vi "Read_FV_Data.vi"(8 "error in (no error)":errorcluster, 9 "RFID":string, 10 "View":bool, 11 "MS SQL Connection":T1) -> (0 "error out":errorcluster, 1 "Enable?":bool, 2 "spreadsheet string":string, 3 "Report":string[][](array[string]), 4 "REsult":T2, 5 "Final View Barcode":string, 6 "All Status":string[](array[string]), 7 "ASR Barcode":string)   [LabVIEW 2020]
uses:
  Controls/FV_Status.ctl
  <vilib>/addons/database/Connection.llb/Conn ObjectReference.ctl
  MS SQL/MS_Global.vi
  <vilib>/ethernetip/ethernetip.llb/EthernetIP Tag Write DINT.vi
  <userlib>/_OpenG.lib/string/string.llb/To Proper Case (String)__ogtk.vi
  <vilib>/addons/database/Connection.llb/Conn Execute.vi
  <vilib>/addons/database/Recordset.llb/Rec Fetch Recordset Data (R).vi
  <vilib>/addons/database/Recordset.llb/Rec Destroy - Connection.vi
  <vilib>/addons/database/_DB Variant To Data/Database Variant To Data.xnode
  <vilib>/addons/database/NI_Database_API.lvlib
  <vilib>/ethernetip/ethernetip.lvlib
panel:
  out "All Result":bool[](array[boolean])
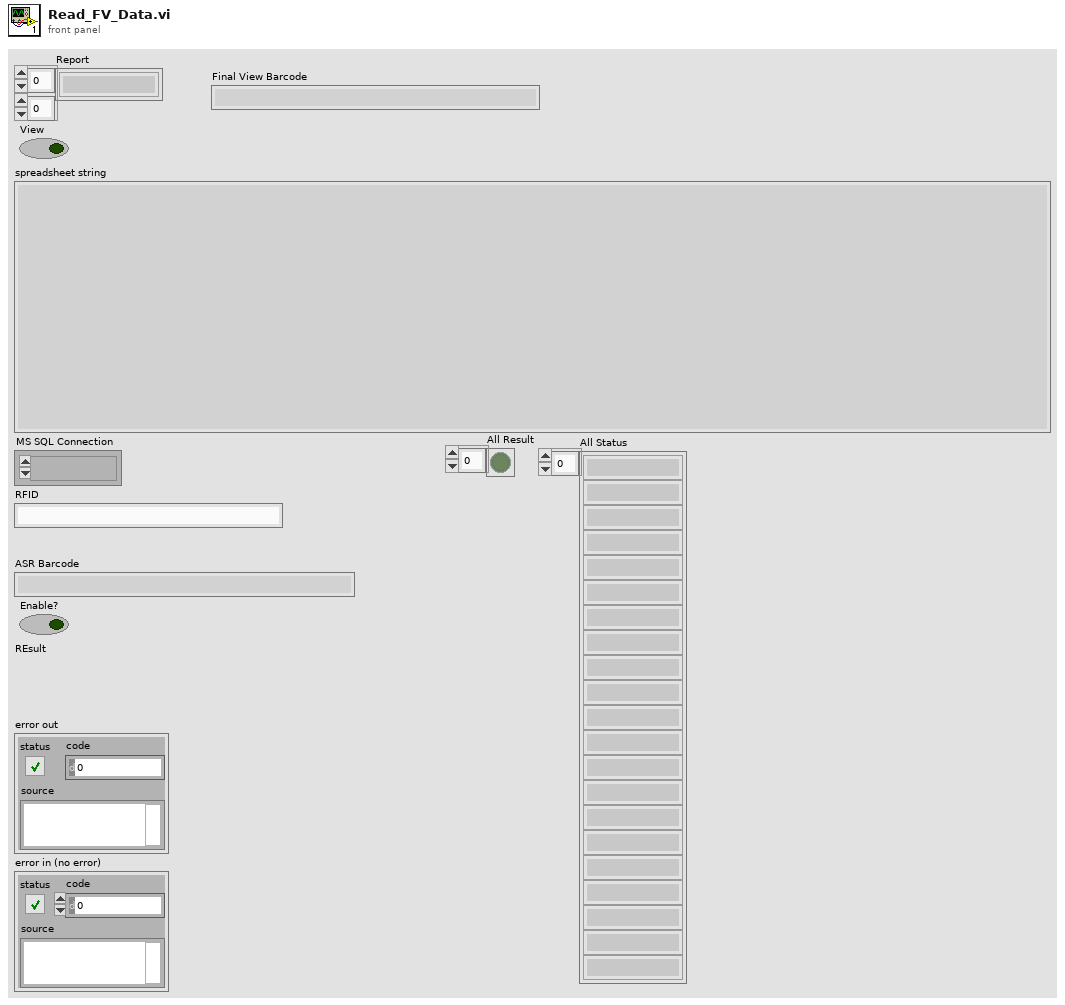
[diagram p1: front panel]
types:
  T1 = typedef "NI_Database_API.lvlib/Conn ObjectReference.ctl" = refnum<k1>
  T2 = typedef "FV_Status.ctl" = u16
  T3 = typedef "TD SQL.ctl" = cluster{"MS SQL Connection":T1, "UDL File":path, "Time":string, "DCODE":string, "WIP+1":i64, "MC No?":i32, "POKAYOKE?":bool, "Expected Result":string, "Result [Status]":string, "Clock":dbl, "RFID":string, "WIP Queue":refnum<queue>, "TS Parameter":T4, "Data_Queue":refnum<queue>[], "RFID Serial No.":string}
  T4 = typedef "TS_Parameter.ctl" = cluster{"ProfitCenterCode":string, "LineCode":string, "WorkOrderNumber":string, "Model":string, "Model_with_Prefix":string, "VendorCode":string, "SetParameterDateCode":string, "PokaYoke":i32, "Target":i32, "Live_DateCode":string, "CustomerPartNumber":string, "Hand":string, "sBarcode":bool, "FCA":i32, "Ent_Stamp":timestamp, "STS_CD":dbl}
  T5 = typedef "NI_Database_API.lvlib/Rec ObjectReference.ctl" = refnum<k1>
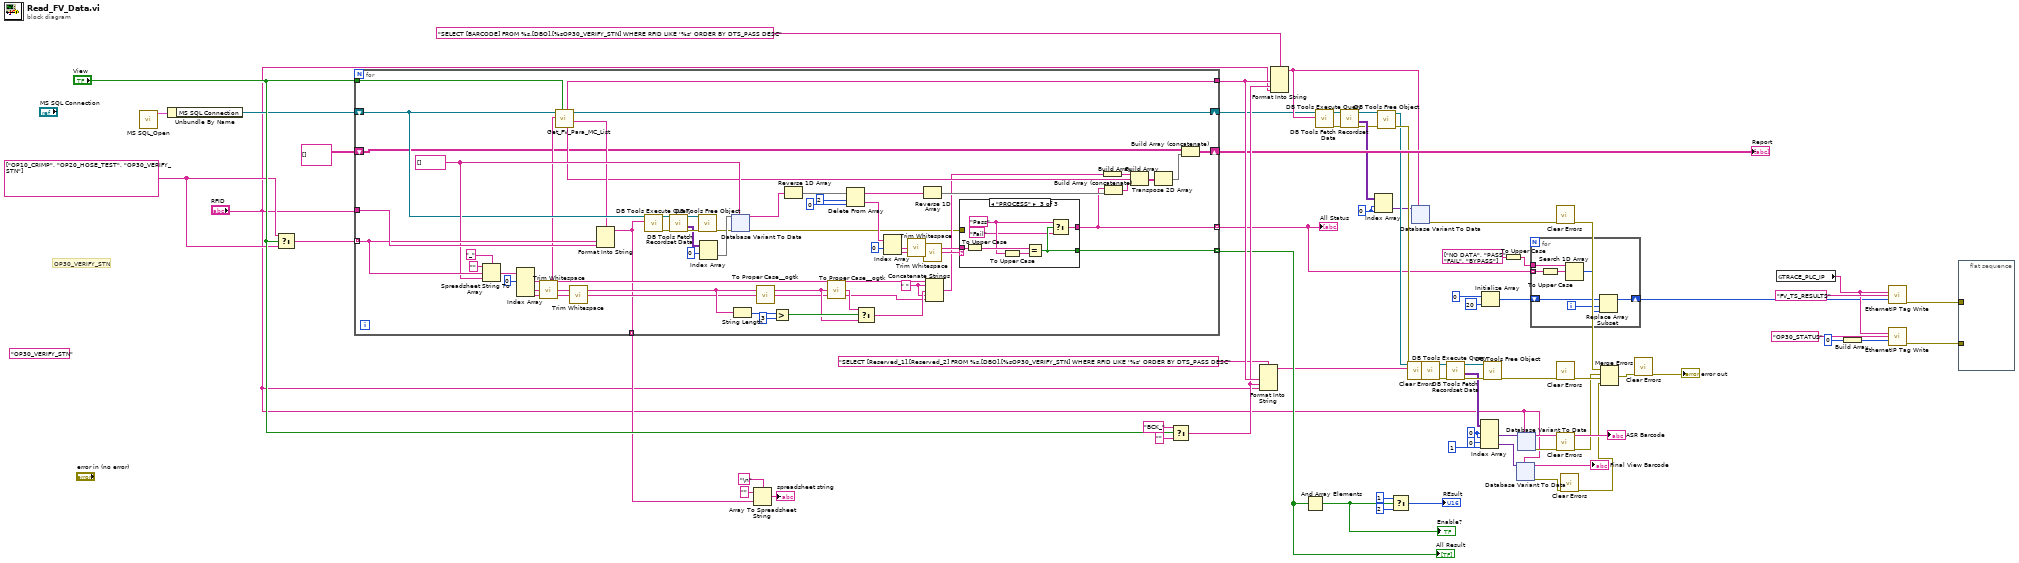
[diagram p0: block diagram]
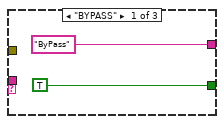
[diagram p2: hidden frame]
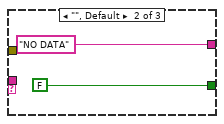
[diagram p3: hidden frame]
diagram:
  w46 = 0 ("index (row)")
  w41 = 0 ("index (row)")
  (unwired) "OP30_VERIFY_STN" ("String")
  w9 = string[] ["OP10_CRIMP", "OP20_HOSE_TEST", "OP30_VERIFY_STN"] ("tables 2")
  # "OP30_VERIFY_STN"
  n1 = call "MS SQL_Open.vi"() -> ("Ref Out"=w10:T3)  [unwired: 9 in, 2 out]
  n2 = Unbundle By Name(w10) -> ("MS SQL Connection"=w28:T1)
  n3 = Select(t=w9, s="View", f=w9) -> (s? t:f=w66:string[])
  n4 = for {
    tunnel: w66 -> [w120] mode=indexing
    tunnel: "RFID" -> [w128]
    tunnel: [w121] -> w57 mode=indexing
    tunnel: [w86] -> w25 mode=indexing
    shift-right: [w102] -> w37
    shift-left: w28 -> [w103]
    tunnel: [w75] -> w60 mode=indexing
    shift-right: [w95] -> w65
    shift-left: string[][] [] ("appended array") -> [w97]
    tunnel: "View" -> [w85]
    tunnel: [w84] -> w72
    w81 = " " ("string")
    w119 = string[] [] ("tables 2")
    n5 = Spreadsheet String To Array(delimiter (Tab)="_", format string="", spreadsheet string=w120, array type (2D Dbl)=w119) -> (array=w112:string[])
    n6 = Index Array(array=w112, index #1=0 ("index")) -> (element #1=w101:string, element #3=w113:string, element #4=w80:string)  [unwired: 3 in, 1 out]
    n7 = call <vilib>:"Trim Whitespace.vi"("string"=w113) -> ("trimmed string"=w107:string)  [unwired: 1 in]
    n8 = call "Get_FV_Para_MC_List.vi"("View"=w85, "Machine No."=w101, "Refnum in"=w103) -> ("Search Queary"=w100:string, "Refnum out"=w102:T1, "Column Display"=w99:string[], "Table"=w84:string)  [unwired: 3 in, 2 out]
    n9 = call <vilib>:"Trim Whitespace.vi"("string"=w80) -> ("trimmed string"=w83:string)  [unwired: 1 in]
    n10 = Format Into String(format string=w100, w120, w128) -> (resulting string=w75:string)  [unwired: 2 in, 1 out]
    n11 = call-poly <vilib>:"DB Tools Execute Query.vi"("SQL query"=w75, "connection reference"=w103) -> ("error out"=w126:errorcluster, "recordset reference"=w127:T5)  [unwired: 6 in]
    n12 = call-poly <vilib>:"DB Tools Fetch Recordset Data.vi"("error in (no error)"=w126, "recordset reference"=w127) -> ("error out"=w78:errorcluster, "recordset data"=w76:variant[][], "recordset reference out"=w79:T5)  [unwired: 3 in]
    n13 = call-poly <vilib>:"DB Tools Free Object.vi"("error in (no error)"=w78, "recordset reference"=w79) -> ("error out"=w73:errorcluster)  [unwired: 8 in, 1 out]
    n14 = Index Array(array=w76, index (row)=0) -> (element=w124:variant[])  [unwired: 1 in]
    n15 = xnode "Database Variant To Data"("database variant"=w124, "error in (no error)"=w73, "type"=w119) -> ("data"=w123:string[], "error out"=w74:errorcluster)
    n16 = String Length(string=w107) -> (length=w111:i32)
    n17 = call-poly <userlib>:"To Proper Case__ogtk.vi"("string"=w83) -> ("proper case string"=w82:string)  [unwired: 4 in]
    n18 = Greater?(x=w111, y=3) -> (0:w109:bool)
    n19 = Reverse 1D Array(array=w123) -> (reversed array=w93:string[])
    n20 = call-poly <userlib>:"To Proper Case__ogtk.vi"("string"=w107) -> ("proper case string"=w108:string)  [unwired: 4 in]
    n21 = Delete From Array(array=w93, length=2, index=0) -> (deleted portion=w91:string[], array with subset deleted=w89:string[])
    n22 = Select(t=w108, s=w109, f=w107) -> (s? t:f=w106:string)
    n23 = Index Array(array=w91, index #1=0 ("index (row)")) -> (element #1=w115:string, element #2=w114:string)  [unwired: 1 in]
    n24 = call <vilib>:"Trim Whitespace.vi"("string"=w115) -> ("trimmed string"=w105:string)  [unwired: 1 in]
    n25 = call <vilib>:"Trim Whitespace.vi"("string"=w114) -> ("trimmed string"=w104:string)  [unwired: 1 in]
    n26 = Reverse 1D Array(array=w89) -> (reversed array=w87:string[])
    n27 = Concatenate Strings(w101, w81, w106, w81, w82) -> (w77:string)
    n28 = case shown="\"PROCESS\"" w104 {
      tunnel: w105 -> [_ _ w139]
      tunnel: [TRUE FALSE w137] -> w121
      tunnel: ["ByPass" ("String") "NO DATA" ("String") w136] -> w86
      tunnel: w74 -> [_ _ _]
      frame "BYPASS" {
      }
      frame "", Default {
      }
      frame "PROCESS" {
        w135 = "Pass" ("y")
        n29 = To Upper Case(1:w139) -> (0:w138:string)
        n30 = To Upper Case(1:w135) -> (0:w133:string)
        n31 = Equal?(x=w138, y=w133) -> (x = y?=w137:bool)
        n32 = Select(t=w135, s=w137, f="Fail" ("t")) -> (s? t:f=w136:string)
      }
    }
    n33 = Build Array(w77) -> (w98:string[])
    n34 = Build Array (concatenate)(w86, w87) -> (w88:string[])
    n35 = Build Array(w98, w99, w88) -> (w96:string[][])
    n36 = Transpose 2D Array(2D array=w96) -> (transposed array=w94:string[][])
    n37 = Build Array (concatenate)(w97, w94) -> (w95:string[][])
  }
  "Report" <- w65
  "All Result" <- w57
  "All Status" <- w25
  n38 = Array To Spreadsheet String(delimiter (Tab)="\n", array=w60, 3:"" ("format string")) -> (spreadsheet string=→"spreadsheet string":string)
  n39 = Select(t="BCK_", s="View", f="") -> (s? t:f=w71:string)
  n40 = Format Into String(format string="SELECT [Reserved_1],[Reserved_2] FROM %s.[DBO].[%sOP30_VERIFY_STN] WHERE RFID LIKE '%s' ORDER BY DTS_PASS DESC" ("String"), w72, w71, "RFID") -> (resulting string=w55:string)  [unwired: 2 in, 1 out]
  n41 = Format Into String(format string="SELECT [BARCODE] FROM %s.[DBO].[%sOP30_VERIFY_STN] WHERE RFID LIKE '%s' ORDER BY DTS_PASS DESC" ("String"), w72, w71, "RFID") -> (resulting string=w44:string)  [unwired: 2 in, 1 out]
  n42 = And Array Elements(Boolean array=w57) -> (logical AND=w18:bool)
  "Enable?" <- w18
  n43 = call-poly <vilib>:"DB Tools Execute Query.vi"("SQL query"=w44, "connection reference"=w37) -> ("error out"=w35:errorcluster, "recordset reference"=w36:T5)  [unwired: 6 in]
  n44 = call-poly <vilib>:"DB Tools Fetch Recordset Data.vi"("error in (no error)"=w35, "recordset reference"=w36) -> ("error out"=w38:errorcluster, "recordset data"=w40:variant[][], "recordset reference out"=w39:T5)  [unwired: 3 in]
  n45 = Index Array(array=w40, index (row)=w41, index (col)=w41) -> (element=w42:variant)
  n46 = call-poly <vilib>:"DB Tools Free Object.vi"("error in (no error)"=w38, "recordset reference"=w39) -> ("error out"=w53:errorcluster, "connection reference"=w52:T1)  [unwired: 8 in]
  n47 = Select(t=T2 1 ("Over all Status"), s=w18, f=T2 2) -> (s? t:f=→"REsult":T2)
  n48 = call <vilib>:"Clear Errors.vi"("error in (no error)"=w53) -> ("error out"=w8:errorcluster)  [unwired: 5 in, 1 out]
  n49 = xnode "Database Variant To Data"("database variant"=w42, "type"=w44) -> ("error out"=w32:errorcluster)  [unwired: 1 in, 1 out]
  n50 = call-poly <vilib>:"DB Tools Execute Query.vi"("error in (no error)"=w8, "SQL query"=w55, "connection reference"=w52) -> ("error out"=w51:errorcluster, "recordset reference"=w50:T5)  [unwired: 5 in]
  n51 = call-poly <vilib>:"DB Tools Fetch Recordset Data.vi"("error in (no error)"=w51, "recordset reference"=w50) -> ("error out"=w49:errorcluster, "recordset data"=w47:variant[][], "recordset reference out"=w48:T5)  [unwired: 3 in]
  n52 = Index Array(array=w47, index (row) #1=w46, index (col) #1=w46, index (row) #2=0 ("index (row)"), index (col) #2=1 ("disabled index (col)")) -> (element #1=w45:variant, element #2=w5:variant)
  n53 = Initialize Array(0 ("index of element"), 20 ("dimension size")) -> (w15:i32[])
  n54 = call-poly <vilib>:"DB Tools Free Object.vi"("error in (no error)"=w49, "recordset reference"=w48) -> ("error out"=w34:errorcluster)  [unwired: 8 in, 1 out]
  n55 = To Upper Case(1:string[] ["NO DATA", "PASS", "FAIL", "BYPASS"] ("Array")) -> (0:w11:string[])
  n56 = xnode "Database Variant To Data"("database variant"=w5, "type"="RFID") -> ("data"=→"Final View Barcode":string, "error out"=w2:errorcluster)  [unwired: 1 in]
  n57 = xnode "Database Variant To Data"("database variant"=w45, "type"="RFID") -> ("data"=→"ASR Barcode":string, "error out"=w33:errorcluster)  [unwired: 1 in]
  n58 = for {
    tunnel: w25 -> [w184] mode=indexing
    shift-right: [w179] -> w14
    shift-left: w15 -> [w182]
    tunnel: w11 -> [w178]
    i -> [w181]
    n59 = To Upper Case(1:w184) -> (0:w183:string)
    n60 = Search 1D Array(1D array=w178, element=w183) -> (index of element=w180:i32)  [unwired: 1 in]
    n61 = Replace Array Subset(array=w182, new element=w180, index=w181) -> (w179:i32[])
  }
  n62 = call <vilib>:"Clear Errors.vi"("error in (no error)"=w32) -> ("error out"=w30:errorcluster)  [unwired: 5 in, 1 out]
  n63 = call <vilib>:"Clear Errors.vi"("error in (no error)"=w34) -> ("error out"=w29:errorcluster)  [unwired: 5 in, 1 out]
  n64 = call <vilib>:"Clear Errors.vi"("error in (no error)"=w33) -> ("error out"=w27:errorcluster)  [unwired: 5 in, 1 out]
  n65 = call <vilib>:"Clear Errors.vi"("error in (no error)"=w2) -> ("error out"=w1:errorcluster)  [unwired: 5 in, 1 out]
  n66 = Merge Errors(w30, w27, w29, w1) -> (w31:errorcluster)
  n67 = call <vilib>:"Clear Errors.vi"("error in (no error)"=w31) -> ("error out"=→"error out":errorcluster)  [unwired: 5 in, 1 out]
  n68 = global read "MS_Global.vi" "TRACE_PLC_IP"() -> (w23:string)
  n69 = Build Array(0 ("element")) -> (w21:i32[])
  n70 = call-poly <vilib>:"EthernetIP Tag Write.vi"("Network Path"=w23, "Tag Name"="FV_TS_RESULTS" ("Network Path"), "Data"=w14) -> ("error out"=w19:errorcluster)  [unwired: 11 in, 1 out]
  n71 = call-poly <vilib>:"EthernetIP Tag Write.vi"("Network Path"=w23, "Tag Name"="OP30_STATUS" ("Network Path"), "Data"=w21) -> ("error out"=w20:errorcluster)  [unwired: 11 in, 1 out]
  n72 = flat-sequence {
    tunnel: w20 -> [_]
    tunnel: w19 -> [_]
    frame #0 {
    }
  }
